vi "checkFinishDirectEnemyPlay.vi"(8 "error in (no error)":errorcluster, 9 "last command_interpreted":T1, 10 "Game":refnum<class "Game.lvclass">, 11 "DirectEnemyPlay in":refnum<class "DirectEnemyPlay.lvclass">) -> (0 "error out":errorcluster, 2 "Boolean":bool, 3 "DirectEnemyPlay out":refnum<class "DirectEnemyPlay.lvclass">)   [LabVIEW 2023, in "DirectEnemyPlay.lvclass"]
uses:
  DirectEnemyPlay.lvclass
  Game_class/Game.lvclass
  Referee_class/command_interpreted.ctl
  Game_class/Game.lvclass/Game.ctl
  Referee_class/Referee.lvclass/Referee.ctl
  Events_class/Events.lvclass/Events.ctl
  Game_class/Read Referee.vi
  Game_class/Read EventsRef.vi
  Game_class/Read EnemyRef.vi
  Events_class/Read ball_out.vi
  Events_class/Read kick.vi
  Events_class/Read touch.vi
  Referee_class/Read command_interpreted.vi
  Referee_class/Referee.lvclass
  Events_class/Events.lvclass
  Enemy_class/Enemy.lvclass
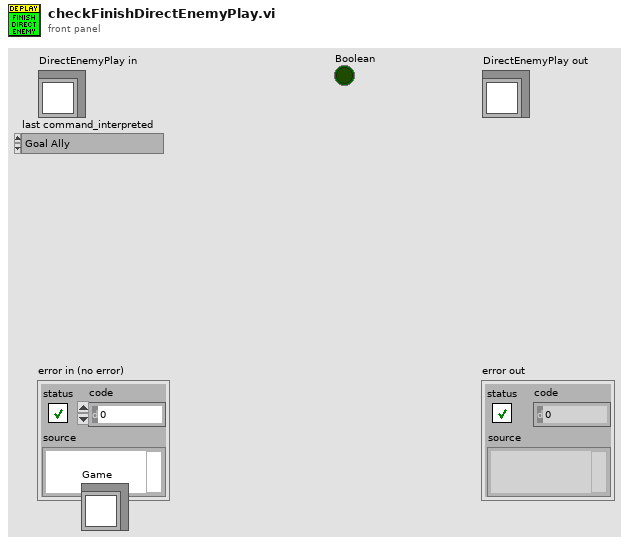
[diagram p1: front panel]
types:
  T1 = typedef "command_interpreted.ctl" = enum16{"Goal Ally", "Goal Enemy", "Ball Placement Enemy", "Ball Placement Ally", "Normal Half Time", "Extra Time  Break", "Extra Half Time", "None", "Post Game", "PKA Normal Start", "Prepare Kickoff Ally", "PKE Normal Start", "Prepare Kickoff Enemy", "Force Start", "Halt", "Timeout", "Prepare Penalty Ally", "Prepare Penalty Enemy", "PPA NormalStart", "PPE Normal Start", "Indirect Free Ally", "Direct Free Enemy", "Direct Free Ally", "Indirect Free Enemy", "Stop"}
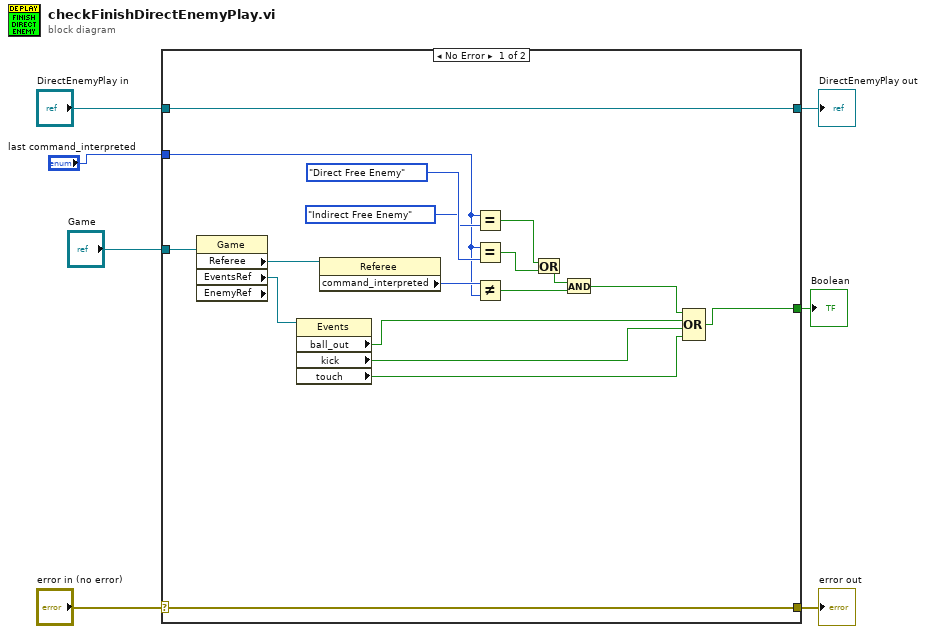
[diagram p0: block diagram]
diagram:
  n1 = case shown="No Error" "error in (no error)" {
    selector: "error in (no error)" -> [w24 w27]
    tunnel: [w24 w27] -> w6
    tunnel: [w25 w26] -> w4
    tunnel: "DirectEnemyPlay in" -> [w25 w26]
    tunnel: "Game" -> [w19 _]
    tunnel: [w15 _] -> w2
    tunnel: "last command_interpreted" -> [w9 _]
    frame No Error {
      n2 = property class="Game" props=["Referee", "EventsRef", "EnemyRef"](reference=w19) -> ("Referee"=w23:refnum<class "Referee.lvclass">, "EventsRef"=w18:refnum<class "Events.lvclass">)  [unwired: 1 in, 3 out]
      n3 = property class="Events"(reference=w18) -> ("ball_out"=w16:bool, "kick"=w14:bool, "touch"=w8:bool)  [unwired: 1 in, 2 out]
      n4 = property class="Referee"(reference=w23) -> ("command_interpreted"=w21:T1)  [unwired: 1 in, 2 out]
      n5 = Equal?(x=w9, y=command_interpreted."Indirect Free Enemy" ("command_interpreted")) -> (x = y?=w11:bool)
      n6 = Equal?(x=w9, y=command_interpreted."Direct Free Enemy" ("command_interpreted")) -> (x = y?=w12:bool)
      n7 = Not Equal?(x=w21, y=w9) -> (x != y?=w20:bool)
      n8 = Or(x=w11, y=w12) -> (x .or. y?=w13:bool)
      n9 = And(x=w13, y=w20) -> (x .and. y?=w17:bool)
      n10 = Compound Arithmetic op=OR(w17, w16, w14, w8) -> (w15:bool)
    }
    frame Error {
    }
  }
  "error out" <- w6
  "DirectEnemyPlay out" <- w4
  "Boolean" <- w2
